vi "API - Add Rx Packet.vi"(8 "error in (no error)":errorcluster, 9 "New Packet ID":i32, 10 "New Packet Name":string, 11 "Item Ref in":T1=18446744073709551615 format="%.0x") -> (0 "error out":errorcluster, 2 "New Packet Ref":T1=18446744073709551615 format="%.0x", 3 "Item Ref Out":T1=18446744073709551615 format="%.0x")   [LabVIEW 2015, in "UDP-Custom-Device System Explorer.lvlib"]
uses:
  UDP-Custom-Device System Explorer.lvlib
  <vilib>/NI Veristand/Custom Device API/Custom Device Item Ref.ctl
  Shared/Constants.vi
  <vilib>/NI Veristand/Custom Device API/Get Item Property (String Array).vi
  <vilib>/NI Veristand/Custom Device API/Set Item Property (String Array).vi
  <vilib>/NI Veristand/Custom Device API/Get Item Property (I32 Array).vi
  <vilib>/NI Veristand/Custom Device API/Set Item Property (I32 Array).vi
  <vilib>/NI VeriStand/Custom Device API/Custom Device API.lvlib
  Shared/UDP-Custom-Device Shared.lvlib
  <vilib>/NI VeriStand/Custom Device Tools/Custom Device Utility Library/Custom Device Utility Library.lvlib
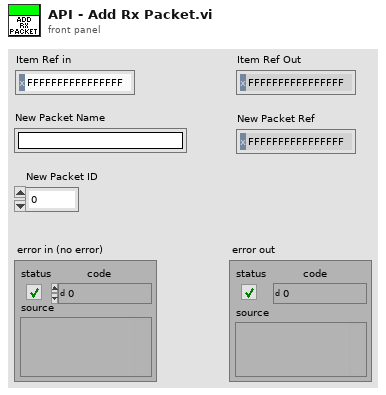
[diagram p1: front panel]
types:
  T1 = typedef "Custom Device API.lvlib/Custom Device Item Ref.ctl" = u64
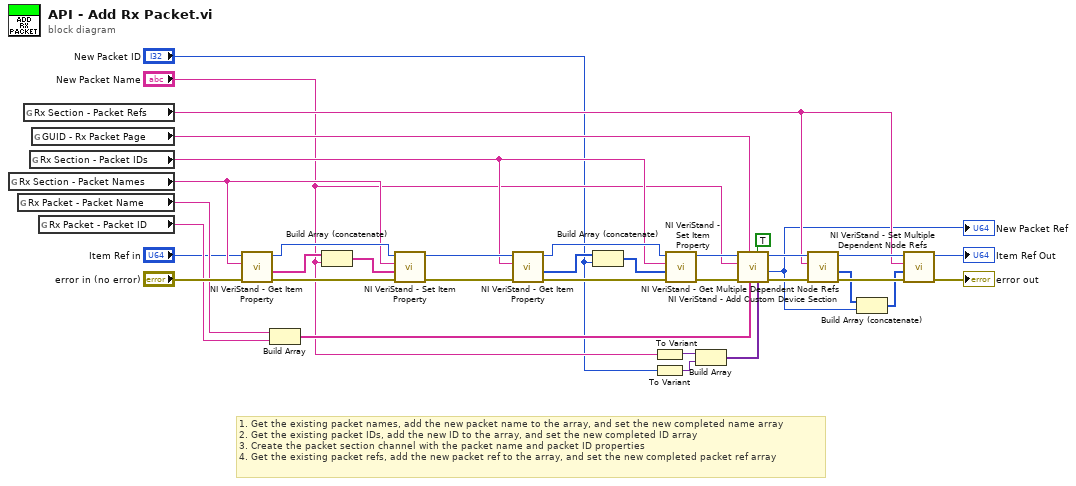
[diagram p0: block diagram]
diagram:
  # "1. Get the existing packet names, add the new packet name to the array, and set the new completed name array\n2. Get the existing packet IDs, add the new ID to the array, and set the new completed ID array\n3. Create the packet section channel with the packet name and packet ID properties\n4. Get the existing packet refs, add the new packet ref to the array, and set the new completed packet ref array"
  n1 = global read "Constants.vi" "Rx Section - Packet Names"() -> (w25:string)
  n2 = global read "Constants.vi" "Rx Packet - Packet Name"() -> (w11:string)
  n3 = global read "Constants.vi" "Rx Section - Packet Refs"() -> (w17:string)
  n4 = global read "Constants.vi" "Rx Section - Packet IDs"() -> (w24:string)
  n5 = global read "Constants.vi" "GUID - Rx Packet Page"() -> (w21:string)
  n6 = global read "Constants.vi" "Rx Packet - Packet ID"() -> (w10:string)
  n7 = call-poly <vilib>:"NI VeriStand - Get Item Property.vi"("error in (no error)"="error in (no error)", "Property Name"=w25, "Item Ref in"="Item Ref in") -> ("error out"=w36:errorcluster, "Value"=w35:string[], "Item Ref out"=w27:T1)  [unwired: 5 in, 1 out]
  n8 = Build Array(w11, w10) -> (w9:string[])
  n9 = Build Array (concatenate)(w35, "New Packet Name") -> (w34:string[])
  n10 = call-poly <vilib>:"NI VeriStand - Set Item Property.vi"("error in (no error)"=w36, "Value"=w34, "Property Name"=w25, "Item Ref in"=w27) -> ("error out"=w30:errorcluster, "Item Ref out"=w29:T1)  [unwired: 5 in, 1 out]
  n11 = call-poly <vilib>:"NI VeriStand - Get Item Property.vi"("error in (no error)"=w30, "Property Name"=w24, "Item Ref in"=w29) -> ("error out"=w31:errorcluster, "Value"=w32:i32[], "Item Ref out"=w26:T1)  [unwired: 5 in, 1 out]
  n12 = Build Array (concatenate)(w32, "New Packet ID") -> (w33:i32[])
  n13 = To Variant(anything="New Packet Name") -> (Variant=w8:variant)
  n14 = To Variant(anything="New Packet ID") -> (Variant=w7:variant)
  n15 = call-poly <vilib>:"NI VeriStand - Set Item Property.vi"("error in (no error)"=w31, "Value"=w33, "Property Name"=w24, "Item Ref in"=w26) -> ("error out"=w28:errorcluster, "Item Ref out"=w23:T1)  [unwired: 5 in, 1 out]
  n16 = Build Array(w8, w7) -> (w6:variant[])
  n17 = call <vilib>:"NI VeriStand - Add Custom Device Section.vi"("Property Values"=w6, "Highlight? (F)"=TRUE, "Property names"=w9, "GUID (Default Section)"=w21, "error in (no error)"=w28, "Section Name"="New Packet Name", "Parent Ref in"=w23) -> ("error out"=w12:errorcluster, "Section Ptr"=w2:T1, "Parent Ref out"=w20:T1)  [unwired: 1 in, 1 out]
  "New Packet Ref" <- w2
  n18 = call <vilib>:"NI VeriStand - Get Multiple Dependent Node Refs.vi"("error in (no error)"=w12, "Base Property Name"=w17, "Item Ref in"=w20) -> ("error out"=w18:errorcluster, "Dependent Node Refs"=w16:T1[], "Item Ref out"=w19:T1)  [unwired: 6 in]
  n19 = Build Array (concatenate)(w16, w2) -> (w15:T1[])
  n20 = call <vilib>:"NI VeriStand - Set Multiple Dependent Node Refs.vi"("error in (no error)"=w18, "Dependent Node Refs"=w15, "Base Property Name"=w17, "Item Ref in"=w19) -> ("error out"=→"error out":errorcluster, "Item Ref out"=→"Item Ref Out":T1)  [unwired: 6 in]
